vi "LoadCustomCursor.vi"(0 "reference in":refnum<class "LcPictureBox.lvclass">, 1 "CustomCusorIndex":u16, 2 "ImageFile":path, 3 "ImageFileContent":string, 5 "error in (no error)":errorcluster) -> (14 "reference out":refnum<class "LcPictureBox.lvclass">, 19 "error out":errorcluster)   [LabVIEW 2020, in "LcPictureBox.lvclass"]
uses:
  LcPictureBox.lvclass
  System.Drawing
  System.Windows.Forms
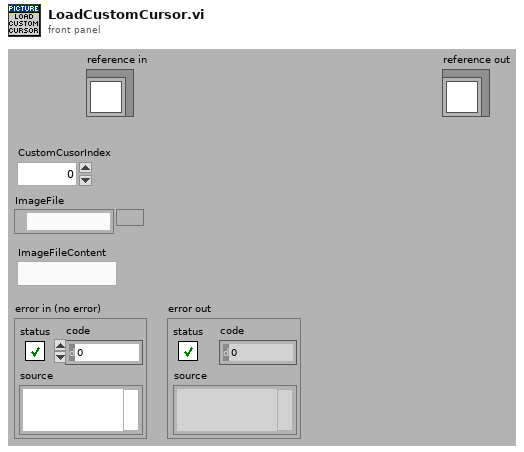
[diagram p1: front panel]
types:
  T1 = typedef "LcPictureBox.lvclass/ObjectAttributes.ctl" = cluster{"PictureBox":refnum<k24>, "ImageSize":cluster{"Width":i32, "Height":i32}, "PenMemory":map{cluster{"Alpha(100%)":dbl, "Color(Black)":u32, "Pen(Width=1, Solid)":T2}, refnum<k24>}, "GraphicsRef":refnum<k24>, "BrushMemory":map{cluster{"Alpha(100%)":dbl, "Color(Black)":u32}, refnum<k24>}, "Images":refnum<k24>[], "ImageIndex":i32, "BgColor(None)":u32, "LoadedImages":map{string, cluster{"ImageOut":refnum<k24>, "ImageSize":cluster{"Width":i32, "Height":i32}}}, "ColorsMemory":map{cluster{"Alpha(100%)":dbl, "Color(Black)":u32}, refnum<k24>}, "CacheSize":i32, "PictureBoxActiveXReference":refnum<vi>, "Scale":dbl, "Offset":cluster{"x":sgl, "y":sgl}, "zoom_center":cluster{"X":i32, "Y":i32}, "ImagesCreated":refnum<k24>[], "CustomCursorImages":map{u16, refnum<k24>}}
  T2 = typedef "LcPictureBox.lvclass/Pen.ctl" = cluster{"Width":u16, "Style":enum32{"Solid", "Dash", "Dot", "DashDot", "DashDotDot"}}
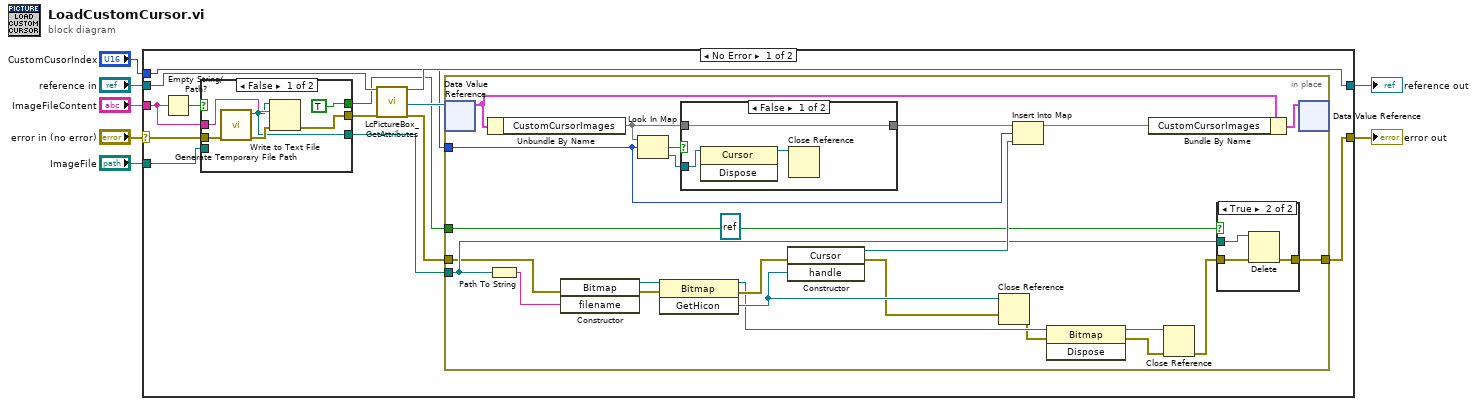
[diagram p0: block diagram]
diagram:
  n1 = case shown="No Error" "error in (no error)" {
    selector: "error in (no error)" -> [w19 w62]
    tunnel: [w9 w62] -> w7
    tunnel: "ImageFileContent" -> [w17 _]
    tunnel: "ImageFile" -> [w18 _]
    tunnel: "reference in" -> [w15 w61]
    tunnel: [w14 w61] -> w2
    tunnel: "CustomCusorIndex" -> [w12 _]
    frame No Error {
      n2 = Empty String/Path?(string/path=w17) -> (empty?=w20:bool)
      n3 = case shown="False" w20 {
        tunnel: w19 -> [w55 w59]
        tunnel: w18 -> [_ w60]
        tunnel: w17 -> [w58 _]
        tunnel: [w56 w59] -> w16
        tunnel: [w54 w60] -> w11
        tunnel: [TRUE _] -> w8
        frame False {
          n4 = call <vilib>:"Generate Temporary File Path.vi"("error in (no error)"=w55) -> ("error out"=w57:errorcluster, "Unique Temporary File Path"=w54:path)  [unwired: 9 in]
          n5 = Write to Text File(file (use dialog)=w54, text=w58, error in=w57) -> (error out=w56:errorcluster)  [unwired: 1 in, 2 out]
        }
        frame True {
        }
      }
      n6 = call "LcPictureBox_GetAttributes.vi"("reference in"=w15, "error in (no error)"=w16) -> ("reference out"=w14:refnum<class "LcPictureBox.lvclass">, "DataRef"=w13:refnum<data-value>, "error out"=w10:errorcluster)  [unwired: 14 in, 1 out]
      n7 = in-place {
        in-place-border: w12 -> [w38]
        in-place-border: w11 -> [w34]
        in-place-border: w10 -> [w28]
        in-place-border: [w33] -> w9
        in-place-border: w8 -> [w35]
        (unwired) refnum<k24> refnum ("handle")
        n8 = in-place-dvr #1(w13) -> (w43:T1)  [unwired: 1 out]
        n9 = Unbundle By Name(w43) -> ("CustomCursorImages"=w40:map{u16, refnum<k24>})
        n10 = Path To String(path=w34) -> (string=w32:string)
        n11 = constructor class="Bitmap"(error in=w28, "filename"=w32) -> (reference out=w31:refnum<k24>, error out=w30:errorcluster)  [unwired: 2 in, 2 out]
        n12 = Look In Map(map=w40, key=w38) -> (key not found?=w41:bool, value=w42:refnum<k24>)  [unwired: 1 in]
        n13 = invoke class="Bitmap" method="GetHicon"(reference=w31, error in=w30) -> (reference out=w24:refnum<k24>, error out=w29:errorcluster, "GetHicon"=w27:refnum<k24>)  [unwired: 1 in]
        n14 = case shown="False" w41 {
          tunnel: w42 -> [w51 _]
          tunnel: w40 -> [w49 w52]
          tunnel: [w49 w52] -> w39
          frame False {
            n15 = invoke class="Cursor" method="Dispose"(reference=w51) -> (reference out=w50:refnum<k24>)  [unwired: 2 in, 2 out]
            n16 = Close Reference(reference=w50) -> ()  [unwired: 1 in, 1 out]
          }
          frame True {
          }
        }
        n17 = constructor class="Cursor"(error in=w29, "handle"=w27) -> (reference out=w36:refnum<k24>, error out=w26:errorcluster)  [unwired: 2 in, 2 out]
        n18 = Close Reference(reference=w27, error in (no error)=w26) -> (error out=w22:errorcluster)
        n19 = Insert Into Map(map in=w39, key=w38, value=w36) -> (map out=w37:map{u16, refnum<k24>})  [unwired: 2 out]
        n20 = invoke class="Bitmap" method="Dispose"(reference=w24, error in=w22) -> (reference out=w23:refnum<k24>, error out=w21:errorcluster)  [unwired: 1 in, 1 out]
        n21 = Bundle By Name(cluster=w43, "CustomCursorImages"=w37) -> (w44:T1)
        n22 = Close Reference(reference=w23, error in (no error)=w21) -> (error out=w25:errorcluster)
        n23 = case shown="True" w35 {
          tunnel: w25 -> [w45 w48]
          tunnel: w34 -> [_ w47]
          tunnel: [w45 w46] -> w33
          frame False {
          }
          frame True {
            n24 = Delete(path (use dialog)=w47, error in=w48) -> (error out=w46:errorcluster)  [unwired: 3 in, 2 out]
          }
        }
        n25 = in-place-dvr #1(w44) -> ()  [unwired: 2 out]
      }
    }
    frame Error {
    }
  }
  "error out" <- w7
  "reference out" <- w2
